vi "RFmxSpecAn CHP (Analysis Only) with Recommended Settings 2.vi"() -> ()   [LabVIEW 2017]
doc: "This example illustrates how to use NI-RFmx in hardware agnostic mode to perform measurements on user provided IQ or Spectrum waveform. The example uses NI-RFSA driver API to acquire waveform from NI RF Signal Analyzer and perform an ACP measurement. The NI-RFSA acquisition settings are read from NI-RFmx session after Commit VI call. The NI-RFmx session is opened with Option String set as \"AnalysisOnly=1\"."
uses:
  <vilib>/Utility/error.llb/DialogType.ctl
  <vilib>/Analysis/NI_AALBase.lvlib
  <vilib>/Analysis/1siggen.llb/Ramp Pattern by Delta.vi
  <vilib>/RFmx/SpecAn/mx/RFmxSpecAn.llb/RFmxSpecAn CHP Fetch Measurement.vi
  <vilib>/RFmx/SpecAn/mx/RFmxSpecAn.llb/RFmxSpecAn TXP Fetch Power Trace.vi
  <vilib>/RFmx/SpecAn/mx/RFmxSpecAn.llb/RFmxSpecAn Analyze (IQ).vi
  <instrlib>/niRFSA/niRFSA.llb/niRFSA Fetch IQ (1D Complex WDT NRec 1Chan).vi
panel:
  in  "Resource Name LO Signal Generation":refnum<k15>="RFSG" caption="resource name"
  in  "Resource Name Test Signal Generation":refnum<k15>="RFSG" caption="resource name"
  in  "Stop Carrier Frequency (Hz)":dbl=6000000000.0 format="%#_6p"
  out "XY Graph":cluster{dbl[], dbl[]}(graph)
  in  "number of records":i64=50
  in  "Start Carrier Frequency (Hz)":dbl=4000000000.0 format="%#_6p"
  in  "Resource Name 2":refnum<k15>="RFSA" caption="Resource Name"
  in  "Reference Level (dBm)":dbl format="%.2f"
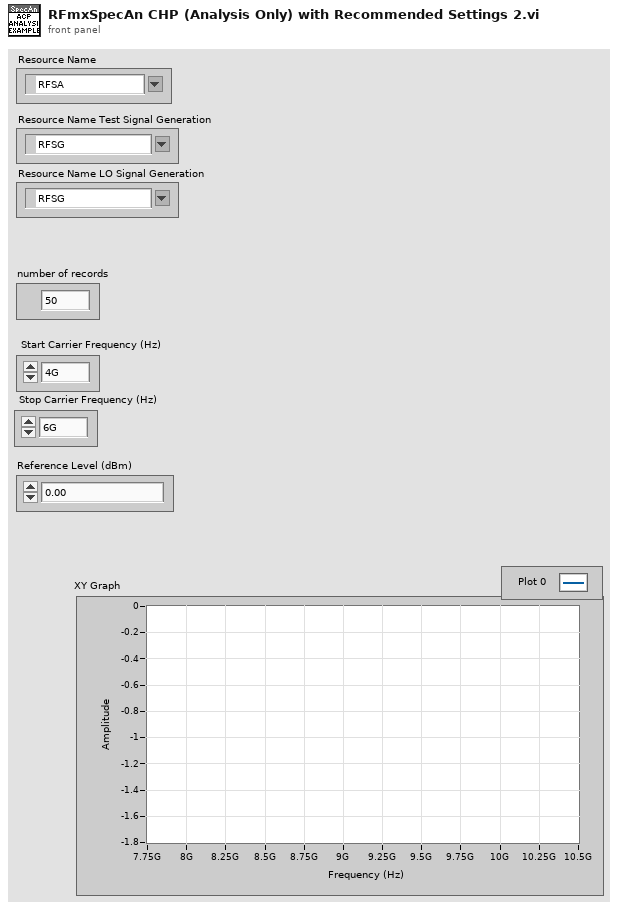
[diagram p1: front panel]
types:
  T1 = typedef "DialogType.ctl" = u16
  T2 = typedef "niRFmx Instrument Handle.ctl" = refnum<k21>
  T3 = enum16{"open", "open or create", "create or replace", "create", "open (read-only)"}
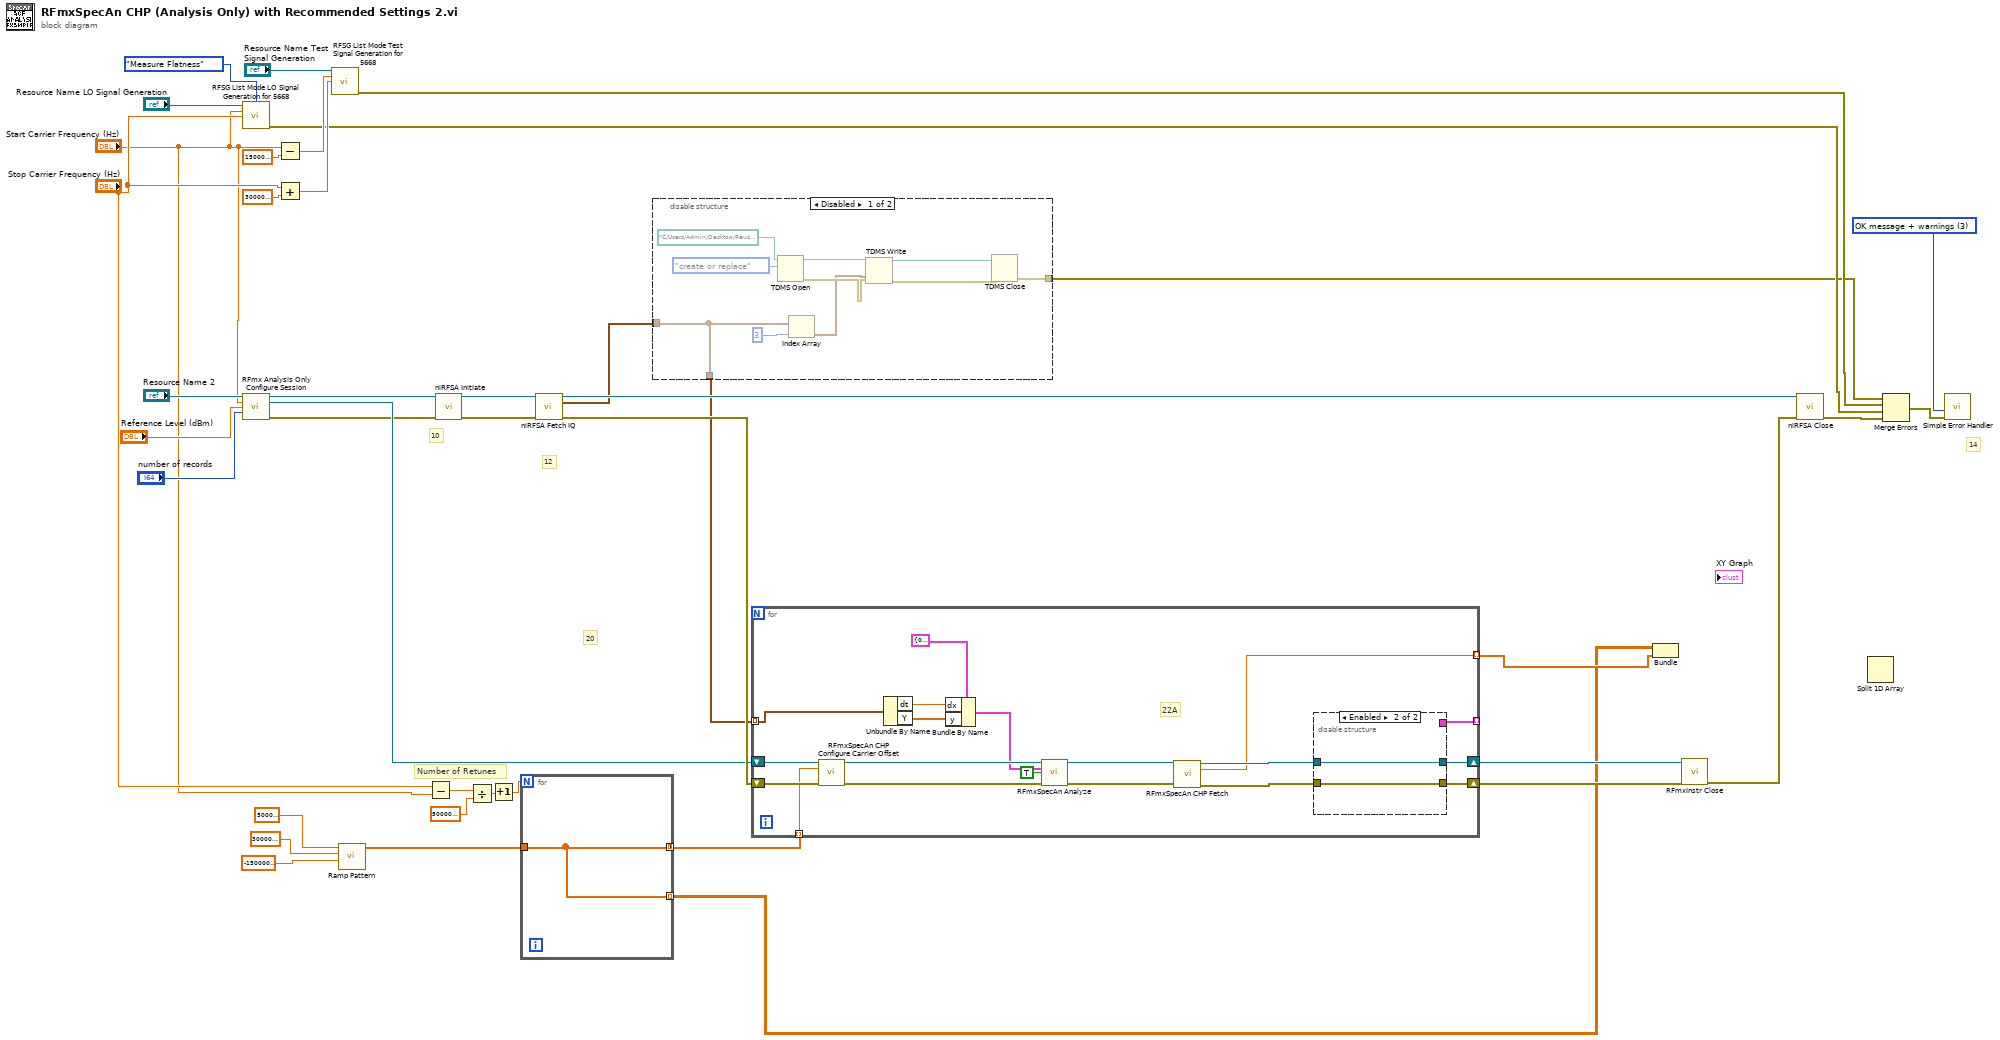
[diagram p0: block diagram]
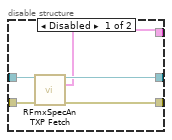
[diagram p3: hidden frame]
diagram:
  w40 = T1 3 items=["no dialog", "OK message", "continue or stop message", "OK message + warnings", "continue/stop + warnings"] ("type of dialog (OK msg:1)")
  # "Number of Retunes"
  # "12"
  # "10"
  # "14"
  # "20"
  n1 = call "RFSG List Mode LO Signal Generation for 5668.vi"("Resource Name"="Resource Name LO Signal Generation", "Mode"=enum16{"Normal", "Measure Flatness"}."Measure Flatness", "Start Frequency"="Start Carrier Frequency (Hz)", "End Frequency"="Stop Carrier Frequency (Hz)") -> ("error out"=w15:errorcluster)  [unwired: 9 in, 2 out]
  n2 = call "RFmx Analysis Only Configure Session.vi"("IVI Refnum in"="Resource Name 2", "Carrier Frequency (Hz)"="Start Carrier Frequency (Hz)", "Reference Level (dBm)"="Reference Level (dBm)", "number of records"="number of records") -> ("RFSA Instrument Handle Out"=w37:refnum<k15>, "RFmx Instrument Handle Out"=w33:T2, "error out 2"=w24:errorcluster)  [unwired: 9 in]
  n3 = Subtract(x="Start Carrier Frequency (Hz)", y=150000000.0) -> (x-y=w21:dbl)
  n4 = Add(x="Stop Carrier Frequency (Hz)", y=300000000.0) -> (x+y=w20:dbl)
  n5 = call "RFSG List Mode Test Signal Generation for 5668.vi"("Resource Name"="Resource Name Test Signal Generation", "Start Frequency"=w21, "End Frequency"=w20) -> ("error out"=w14:errorcluster)  [unwired: 11 in, 1 out]
  n6 = call-poly <vilib>:"Ramp Pattern.vi"("start"=-150000000.0, "end"=300000000.0, "delta"=50000000.0) -> ("Ramp Pattern"=w6:dbl[])  [unwired: 6 in, 2 out]
  n7 = Subtract(x="Stop Carrier Frequency (Hz)", y="Start Carrier Frequency (Hz)") -> (x-y=w12:dbl)
  n8 = call <instrlib>:"niRFSA Initiate.vi"("instrument handle"=w37, "error in"=w24) -> ("instrument handle out"=w32:refnum<k15>, "error out"=w31:errorcluster)  [unwired: 12 in]
  n9 = Divide(x=w12, y=500000000.0) -> (x/y=w10:dbl)
  n10 = Increment(x=w10) -> (x+1=w9:dbl)
  n11 = for {
    N: w9 -> [_]
    tunnel: w6 -> [w42]
    tunnel: [w42] -> w7 mode=concatenating
    tunnel: [w42] -> w4 mode=indexing
  }
  n12 = call-poly <instrlib>:"niRFSA Fetch IQ.vi"("instrument handle"=w32, "error in"=w31) -> ("instrument handle out"=w39:refnum<k15>, "data"=w2:waveform(cdb)[], "error out"=w36:errorcluster)  [unwired: 11 in]
  n13 = disable-structure shown="Disabled" {
    disable-tunnel: [w46 _] -> w3
    disable-tunnel: w2 -> [w43 w53]
    disable-tunnel: [w43 w53] -> w1
    frame Disabled {
      n14 = TDMS Open(10:T3."create or replace" ("operation (0:open)"), 11:path "C:/Users/Admin/Desktop/Reuse/Scanning Speed PXIe 5668/Data8G.tdms.txt" ("file path")) -> (0:w50:errorcluster, 3:w49:refnum<k34>)  [unwired: 5 in]
      n15 = Index Array(array=w43, index=3) -> (element=w44:waveform(cdb))
      n16 = TDMS Write(0:w49, 9:w44, 11:w50) -> (4:w47:refnum<k34>, 15:w48:errorcluster)  [unwired: 3 in, 2 out]
      n17 = TDMS Close(8:w48, 11:w47) -> (0:w46:errorcluster)  [unwired: 1 out]
    }
    frame Enabled {
    }
  }
  n18 = for {
    shift-right: [w70] -> w34
    shift-left: w36 -> [w72]
    shift-right: [w71] -> w35
    shift-left: w33 -> [w59]
    tunnel: [w60] -> w27 mode=indexing
    tunnel: w1 -> [w58] mode=indexing
    tunnel: [w67] -> _ mode=indexing
    tunnel: w7 -> [w61] mode=indexing
    # "22A"
    n19 = call <vilib>:"RFmxSpecAn CHP Configure Carrier Offset.vi"("Instrument Handle In"=w59, "Carrier Frequency (Hz)"=w61, "error in (no error)"=w72) -> ("Instrument Handle Out"=w62:refnum<k21>, "error out"=w63:errorcluster)  [unwired: 11 in]
    n20 = Unbundle By Name(w58) -> ("dt"=w56:dbl, "Y"=w55:cdb[])
    n21 = Bundle By Name(cluster=cluster{"x0":dbl, "dx":dbl, "y":csg[]} {"x0"=0.0, "dx"=0.0, "y"=[]} ("IQ"), "dx"=w56, "y"=w55) -> (w54:cluster{"x0":dbl, "dx":dbl, "y":csg[]})
    n22 = call-poly <vilib>:"RFmxSpecAn Analyze.vi"("Instrument Handle In"=w62, "IQ"=w54, "Reset?"=TRUE, "error in (no error)"=w63) -> ("Instrument Handle Out"=w66:refnum<k21>, "error out"=w65:errorcluster)  [unwired: 8 in, 2 out]
    n23 = call-poly <vilib>:"RFmxSpecAn CHP Fetch.vi"("Instrument Handle In"=w66, "error in (no error)"=w65) -> ("Instrument Handle Out"=w64:refnum<k21>, "Absolute Power (dBm)"=w60:dbl, "error out"=w68:errorcluster)  [unwired: 8 in, 3 out]
    n24 = disable-structure shown="Enabled" {
      disable-tunnel: [w77 w79] -> w71
      disable-tunnel: [w76 w78] -> w70
      disable-tunnel: w68 -> [w75 w78]
      disable-tunnel: [w74 _] -> w67
      disable-tunnel: w64 -> [w73 w79]
      frame Disabled {
        n25 = call-poly <vilib>:"RFmxSpecAn TXP Fetch.vi"("Instrument Handle In"=w73, "error in (no error)"=w75) -> ("Instrument Handle Out"=w77:refnum<k21>, "Power (dBm)"=w74:cluster{"x0":dbl, "dx":dbl, "y":sgl[]}, "error out"=w76:errorcluster)  [unwired: 11 in]
      }
      frame Enabled {
      }
    }
  }
  n26 = Bundle("Ramp Pattern"=w4, w27) -> ()  [unwired: 1 in, 1 out]
  n27 = call <vilib>:"RFmxInstr Close.vi"("Instrument Handle In"=w35, "error in (no error)"=w34) -> ("error out"=w41:errorcluster)  [unwired: 13 in]
  n28 = call <instrlib>:"niRFSA Close.vi"("instrument handle"=w39, "error in"=w41) -> ("error out"=w16:errorcluster)  [unwired: 13 in]
  n29 = Split 1D Array() -> ()  [unwired: 2 in, 2 out]
  n30 = Merge Errors(w3, w14, w15, w16) -> (w13:errorcluster)
  n31 = call <vilib>:"Simple Error Handler.vi"("type of dialog (OK msg:1)"=w40, "error in (no error)"=w13) -> ()  [unwired: 3 in, 5 out]
